vi "_decode_STB.vi"(8 "Compose Summary string (F)":bool, 11 "STB in":u16 format="%.0x") -> (0 "Summary string":string, 1 "Error":bool, 2 "OPC (ESB)":bool, 3 "MAV":bool)   [LabVIEW 2020, in "Rohde&Schwarz RTx Oscilloscopes.lvlib" / "rsidr_core.lvlib"]
uses:
  rsidr_core.lvlib
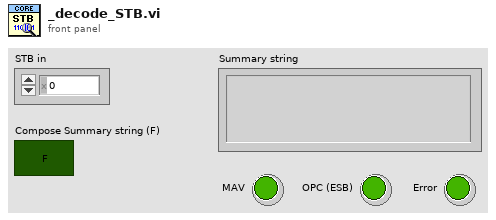
[diagram p1: front panel]
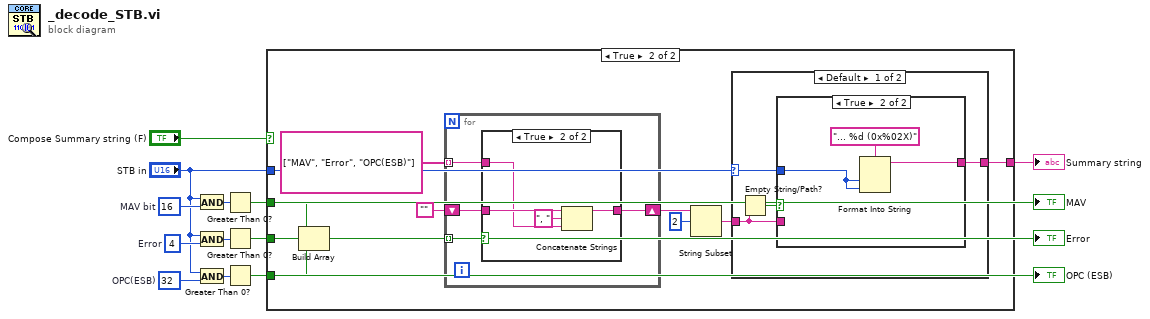
[diagram p0: block diagram]
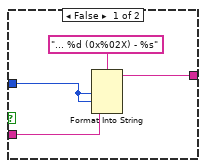
[diagram p3: hidden frame]
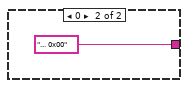
[diagram p4: hidden frame]
diagram:
  w7 = u16 32  # OPC(ESB)
  w10 = u16 4  # Error
  w11 = u16 16  # MAV bit
  n1 = And(x="STB in", y=w11) -> (x .and. y?=w12:u16)
  n2 = And(x="STB in", y=w10) -> (x .and. y?=w9:u16)
  n3 = And(x="STB in", y=w7) -> (x .and. y?=w8:u16)
  n4 = Greater Than 0?(x=w12) -> (x > 0?=w5:bool)
  "MAV" <- w5
  n5 = Greater Than 0?(x=w9) -> (x > 0?=w4:bool)
  "Error" <- w4
  n6 = Greater Than 0?(x=w8) -> (x > 0?=w3:bool)
  "OPC (ESB)" <- w3
  n7 = case shown="True" "Compose Summary string (F)" {
    tunnel: w5 -> [_ w23]
    tunnel: w4 -> [_ w22]
    tunnel: w3 -> [_ w21]
    tunnel: [_ w14] -> w2
    tunnel: "STB in" -> [_ w13]
    frame False {
    }
    frame True {
      n8 = Build Array(w23, w22, w21) -> (w20:bool[])
      n9 = for {
        tunnel: w20 -> [w39] mode=indexing
        shift-right: [w36] -> w17
        shift-left: "" ("Empty String Constant") -> [w38]
        tunnel: string[] ["MAV", "Error", "OPC(ESB)"] -> [w37] mode=indexing
        n10 = case shown="True" w39 {
          tunnel: w38 -> [w40 w44]
          tunnel: w37 -> [_ w42]
          tunnel: [w40 w41] -> w36
          frame False {
          }
          frame True {
            n11 = Concatenate Strings(w44, ", " ("string"), w42) -> (w41:string)
          }
        }
      }
      n12 = String Subset(string=w17, offset (0)=2) -> (substring=w15:string)  [unwired: 1 in]
      n13 = case shown="Default" w13 {
        selector: w13 -> [w26 _]
        tunnel: w15 -> [w25 _]
        tunnel: [w27 "... 0x00" ("String to write")] -> w14
        frame Default {
          n14 = Empty String/Path?(string/path=w25) -> (empty?=w24:bool)
          n15 = case shown="True" w24 {
            tunnel: w25 -> [w30 _]
            tunnel: [w29 w33] -> w27
            tunnel: w26 -> [w28 w32]
            frame False {
              n16 = Format Into String(format string="... %d (0x%02X) - %s" ("String to write"), w28, w28, w30) -> (resulting string=w29:string)  [unwired: 2 in, 1 out]
            }
            frame True {
              n17 = Format Into String(format string="... %d (0x%02X)" ("String to write"), w32, w32) -> (resulting string=w33:string)  [unwired: 2 in, 1 out]
            }
          }
        }
        frame 0 {
        }
      }
    }
  }
  "Summary string" <- w2
